vi "Read Msg Output.vi"(10 "Msg Output":refnum<class "Msg Output.lvclass">) -> ()   [LabVIEW 2025, in "jettl.lvlib" / "Stop Msg.lvlib" / "Stop Msg Output.lvclass"]
uses:
  Stop Msg Output.lvclass
  Msg Output/Msg Output.lvclass
  Stop Msg Output.lvclass/Stop Msg Output.ctl
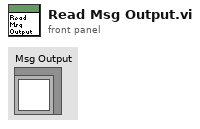
[diagram p1: front panel]
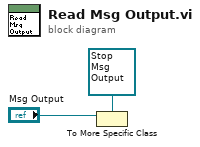
[diagram p0: block diagram]
diagram:
  n1 = To More Specific Class(target class=refnum<class "Stop Msg Output.lvclass"> refnum ("jettl.lvlib:Stop Msg.lvlib:Stop Msg Output.lvclass"), reference="Msg Output") -> ()  [unwired: 1 in, 2 out]
